vi "Power_Meter.vi"() -> ()   [LabVIEW 2009]
panel:
  in  "Timer (mS)":u32=1000
  in  "stop":bool
  out "Power returned (dBm)":dbl(graph)=-47.6902031
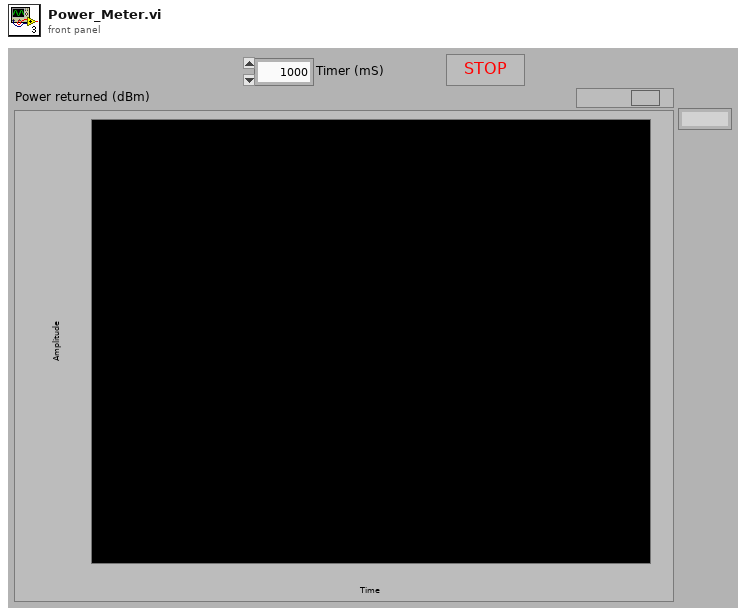
[diagram p1: front panel]
types:
  T1 = enum16{"N1911A", "Siggen", "34980a", "E4418B", "Rvp8"}
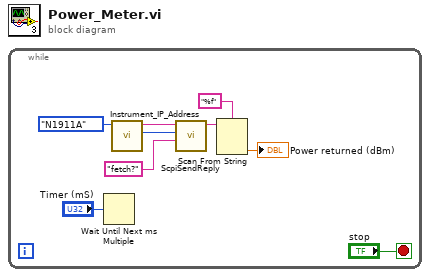
[diagram p0: block diagram]
diagram:
  n1 = while {
    stop <- "stop" stop-if-true
    n2 = Wait Until Next ms Multiple(millisecond multiple="Timer (mS)") -> ()  [unwired: 1 out]
    n3 = call "Instrument_IP_Address.vi"("Instrument"=T1."N1911A") -> ("Port"=w3:u16, "IP Address"=w4:string)  [unwired: 9 in]
    n4 = call "ScpiSendReply.vi"("Command"="fetch?" ("format string"), "TCP port"=w3, "IP Address"=w4) -> ("Reply"=w8:string)  [unwired: 6 in, 1 out]
    n5 = Scan From String(format string="%f", input string=w8) -> (output 1=→"Power returned (dBm)":dbl)  [unwired: 3 in, 3 out]
  }
